vi "Shutdown.vi"(8 "error in (no error)":errorcluster, 11 "Assembler in":refnum<class "Assembler.lvclass">) -> (0 "error out":errorcluster)   [LabVIEW 2019, in "TimingDRV Engine.lvlib" / "Assembler.lvclass"]
uses:
  Assembler.lvclass
  Assembler.lvclass/Assembler.ctl
  Parent Classes/Process/Process.lvclass
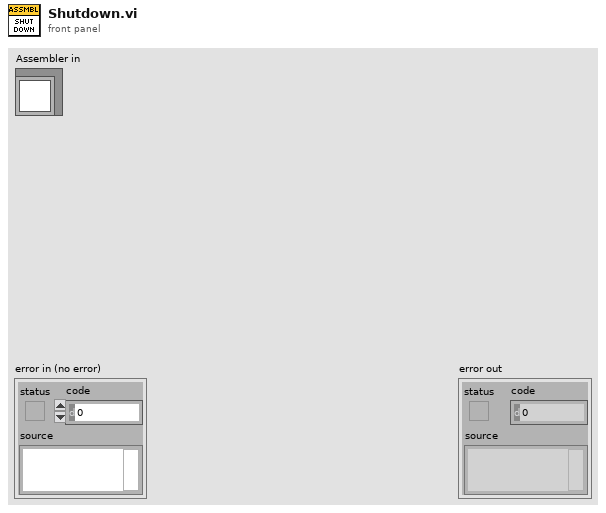
[diagram p1: front panel]
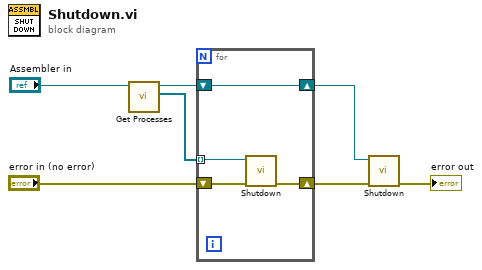
[diagram p0: block diagram]
diagram:
  n1 = call "Get Processes.vi"("Assembler in"="Assembler in") -> ("Processes"=w4:refnum<class "Process.lvclass">[], "Assembler out"=w3:refnum<class "Assembler.lvclass">)  [unwired: 9 in]
  n2 = for {
    tunnel: w4 -> [w10] mode=indexing
    shift-right: [w9] -> w1
    shift-left: w3 -> [w9]
    shift-right: [w8] -> w2
    shift-left: "error in (no error)" -> [w11]
    n3 = call-dynamic "Shutdown.vi"("error in (no error)"=w11, "Process in"=w10) -> ("error out"=w8:errorcluster)  [unwired: 9 in]
  }
  n4 = call-parent "Shutdown.vi"("error in (no error)"=w2, "Process in"=w1) -> ("error out"=→"error out":errorcluster)  [unwired: 9 in]
